vi "LowpassFilter.vi"(8 "ln_k":dbl, 10 "Ts":dbl, 11 "Tf":dbl) -> (3 "Filter output":dbl)   [LabVIEW 2018]
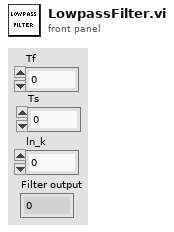
[diagram p1: front panel]
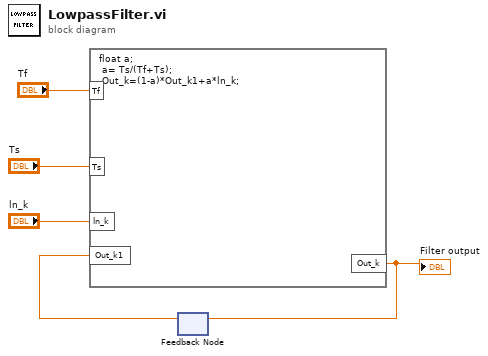
[diagram p0: block diagram]
diagram:
  n1 = feedback #1() -> (w1:dbl)  [unwired: 1 in]
  n2 = formula code="float a;\n a= Ts/(Tf+Ts);\n Out_k=(1-a)*Out_k1+a*ln_k;"("Tf"="Tf", "Ts"="Ts", "ln_k"="ln_k", "Out_k1"=w1) -> ("Out_k"=w2:dbl)
  "Filter output" <- w2
  n3 = feedback-in #1(w2) -> ()
